vi "modbusTCPMasterDriver.vi"(6 "Modbus Driver Selector Enum":T4, 8 "Error In":errorcluster, 9 "Read Modbus Register":T1, 10 "Write Single Register Modbus":T2, 11 "Open Modbus Connection Cluster":T3) -> (0 "Error Out":errorcluster, 3 "Register Value":u16[](array[numeric]))   [LabVIEW 2018]
uses:
  controls/modbusDriverSelectorEnum.ctl
  controls/openModbusConnectionCluster.ctl
  controls/writeSingleRegisterModbusCluster.ctl
  controls/readRegisterModbusCluster.ctl
  <vilib>/NI/Modbus Library/API/Master/Modbus Master.lvclass
  C:/Program Files (x86)/National Instruments/LabVIEW 2018/vi.lib/NI/Modbus Library/API/Modbus API.lvclass
  <vilib>/NI/Modbus Library/API/Wrapper/Create TCP Master.vi
  <vilib>/NI/Modbus Library/API/Modbus API.lvclass
  <vilib>/NI/Modbus Library/API/Wrapper/API Main.lvlib
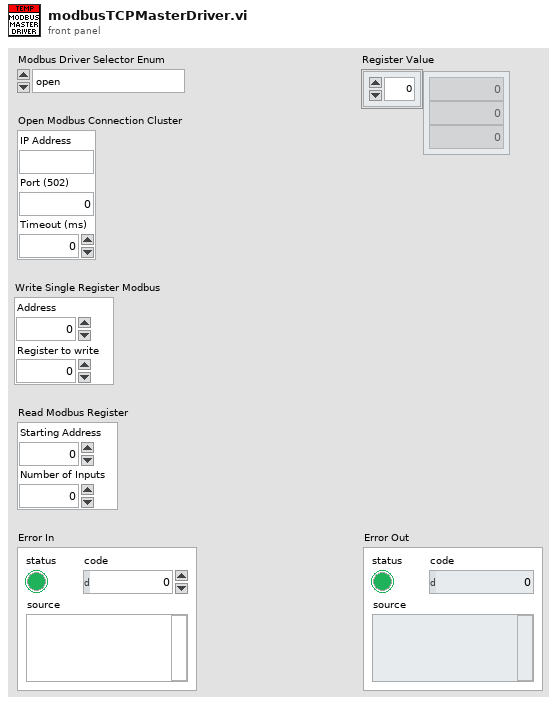
[diagram p1: front panel]
types:
  T1 = typedef "readRegisterModbusCluster.ctl" = cluster{"Starting Address":u16, "Number of Inputs":u16}
  T2 = typedef "writeSingleRegisterModbusCluster.ctl" = cluster{"Address":u16, "Register to write":u16}
  T3 = typedef "openModbusConnectionCluster.ctl" = cluster{"IP Address":string, "Timeout (ms)":i32, "Port (502)":u16}
  T4 = typedef "modbusDriverSelectorEnum.ctl" = enum16{"open", "write single holding registers", "read holding registers", "close"}
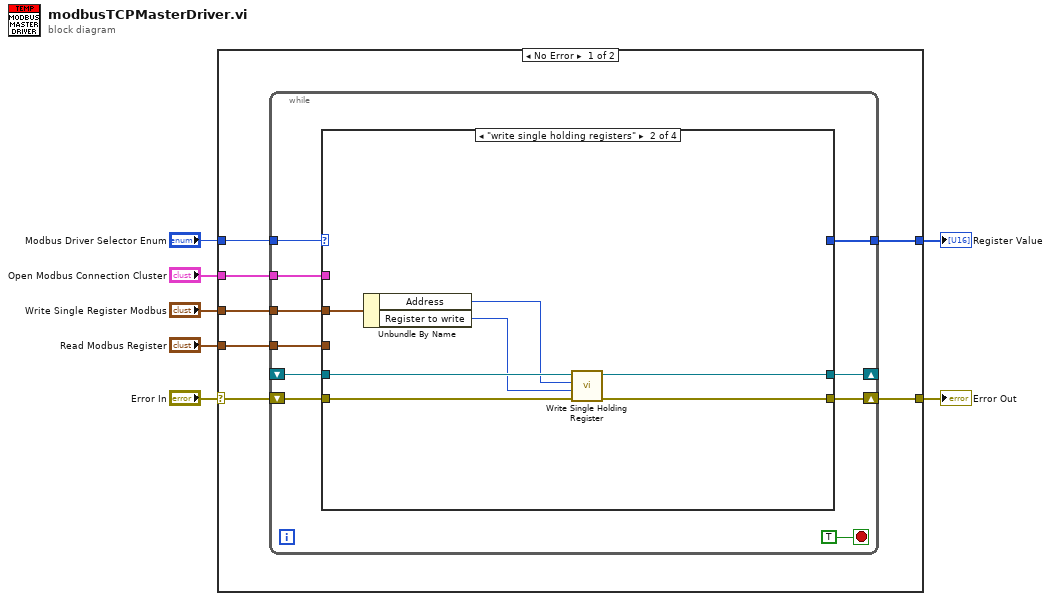
[diagram p0: block diagram]
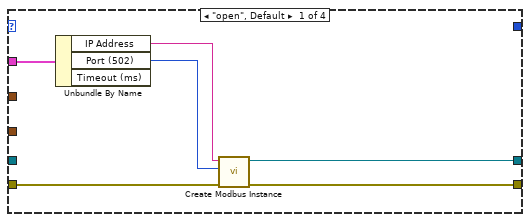
[diagram p2: hidden frame]
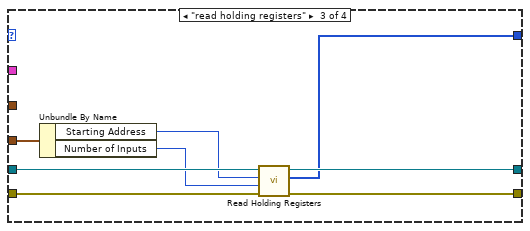
[diagram p3: hidden frame]
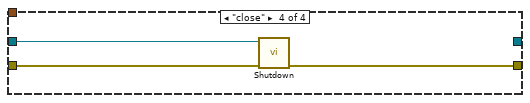
[diagram p4: hidden frame]
diagram:
  n1 = case shown="No Error" "Error In" {
    selector: "Error In" -> [w14 w49]
    tunnel: [w13 w49] -> w5
    tunnel: "Modbus Driver Selector Enum" -> [w12 _]
    tunnel: [w11 _] -> w4
    tunnel: "Read Modbus Register" -> [w10 _]
    tunnel: "Write Single Register Modbus" -> [w9 _]
    tunnel: "Open Modbus Connection Cluster" -> [w8 _]
    frame No Error {
      n2 = while {
        tunnel: w12 -> [w22]
        shift-right: [w23] -> w13
        shift-left: w14 -> [w24]
        shift-right: [w21] -> _
        shift-left: _ -> [w20]
        tunnel: [w18] -> w11
        tunnel: w10 -> [w17]
        tunnel: w9 -> [w16]
        tunnel: w8 -> [w15]
        stop <- TRUE stop-if-true
        n3 = case shown="\"write single holding registers\"" w22 {
          tunnel: w24 -> [w30 w36 w44 w47]
          tunnel: [w27 w37 w45 w48] -> w23
          tunnel: [w29 w35 w43 _] -> w21
          tunnel: w20 -> [_ w34 w42 w46]
          tunnel: [_ _ w41 _] -> w18
          tunnel: w17 -> [_ _ w40 _]
          tunnel: w16 -> [_ w33 _ _]
          tunnel: w15 -> [w28 _ _ _]
          frame "open", Default {
            n4 = Unbundle By Name(w28) -> ("IP Address"=w26:string, "Port (502)"=w25:u16)  [unwired: 1 out]
            n5 = call-poly <vilib>:"Create Modbus Instance.vi"("error in"=w30, "port (502)"=w25, "address"=w26) -> ("error out"=w27:errorcluster, "TCP master instance"=w29:refnum<class "Modbus Master.lvclass">)  [unwired: 7 in]
          }
          frame "write single holding registers" {
            n6 = Unbundle By Name(w33) -> ("Address"=w32:u16, "Register to write"=w31:u16)
            n7 = call-dynamic "Write Single Holding Register.vi"("error in"=w36, "register to write"=w31, "address"=w32, "Modbus instance in"=w34) -> ("error out"=w37:errorcluster, "Modbus instance out"=w35:refnum<class "Modbus API.lvclass">)  [unwired: 6 in]
          }
          frame "read holding registers" {
            n8 = Unbundle By Name(w40) -> ("Starting Address"=w39:u16, "Number of Inputs"=w38:u16)
            n9 = call-dynamic "Read Holding Registers.vi"("error in"=w44, "number of inputs"=w38, "starting address"=w39, "Modbus instance in"=w42) -> ("error out"=w45:errorcluster, "register values"=w41:u16[], "Modbus instance out"=w43:refnum<class "Modbus API.lvclass">)  [unwired: 5 in]
          }
          frame "close" {
            n10 = call-dynamic "Shutdown.vi"("error in"=w47, "Modbus instance in"=w46) -> ("error out"=w48:errorcluster)  [unwired: 9 in]
          }
        }
      }
    }
    frame Error {
    }
  }
  "Error Out" <- w5
  "Register Value" <- w4
